vi "read.vi"(8 "error in (no error)":errorcluster, 10 "ILC":refnum<class "ILC.lvclass">, 11 "ReadILCLIMSW1Strategy in":refnum<class "ReadILCDCAPressure2Strategy.lvclass">) -> (0 "error out":errorcluster, 2 "Value":dbl, 3 "ReadILCLIMSW1Strategy out":refnum<class "ReadILCDCAPressure2Strategy.lvclass">)   [LabVIEW 2015, in "ReadILCDCAPressure2Strategy.lvclass"]
uses:
  ReadILCDCAPressure2Strategy.lvclass
  <userlib>/Common/ILC/ILC/ILC.lvclass
  <userlib>/Common/ILC/ILC/ILC.lvclass/ILC.ctl
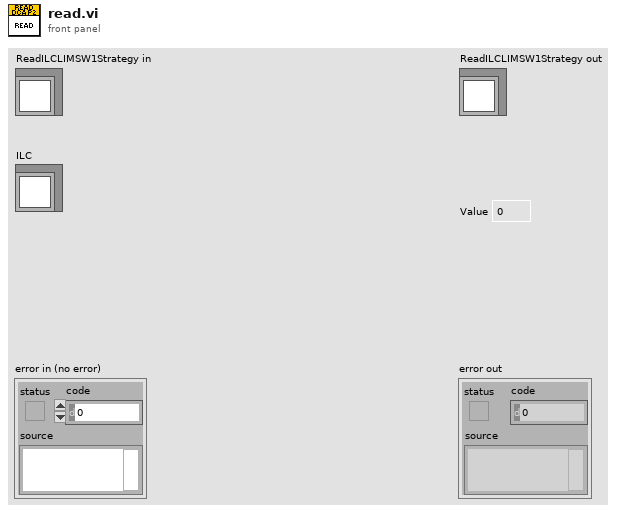
[diagram p1: front panel]
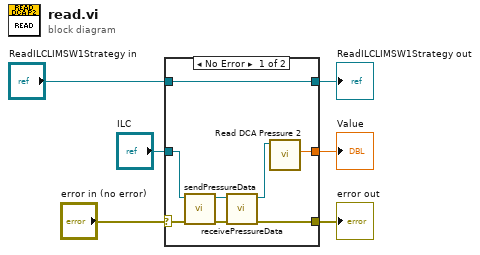
[diagram p0: block diagram]
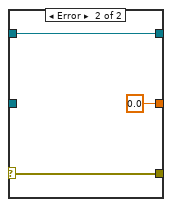
[diagram p2: hidden frame]
diagram:
  n1 = case shown="No Error" "error in (no error)" {
    selector: "error in (no error)" -> [w9 w17]
    tunnel: [w7 w17] -> w5
    tunnel: [w14 w16] -> w3
    tunnel: "ReadILCLIMSW1Strategy in" -> [w14 w16]
    tunnel: [w13 0.0 ("Value")] -> w2
    tunnel: "ILC" -> [w10 _]
    frame No Error {
      n2 = call <userlib>:"sendPressureData.vi"("error in (no error)"=w9, "ILC in"=w10) -> ("error out"=w8:errorcluster, "ILC out"=w12:refnum<class "ILC.lvclass">)  [unwired: 8 in]
      n3 = call <userlib>:"receivePressureData.vi"("error in (no error)"=w8, "ILC in"=w12) -> ("error out"=w7:errorcluster, "ILC out"=w11:refnum<class "ILC.lvclass">)  [unwired: 8 in]
      n4 = call <userlib>:"Read DCA Pressure 2.vi"("ILC in"=w11) -> ("DCA Pressure 2"=w13:dbl)  [unwired: 9 in, 1 out]
    }
    frame Error {
    }
  }
  "error out" <- w5
  "ReadILCLIMSW1Strategy out" <- w3
  "Value" <- w2
